vi "Send Image Data.vi"(4 "error in (no error)":errorcluster, 6 "image data":T1, 7 "Response Notifier":string) -> (0 "error out":errorcluster)   [LabVIEW 2020, in "Startup Processes.lvlib"]
uses:
  Startup Processes.lvlib
  <vilib>/picture/picture.llb/imagedata.ctl
  <vilib>/Utility/sysdir.llb/System Directory Type.ctl
  toolbox/Standard Signalling/not_Generic Named Notifier/not_Generic Named Notifier.lvlib
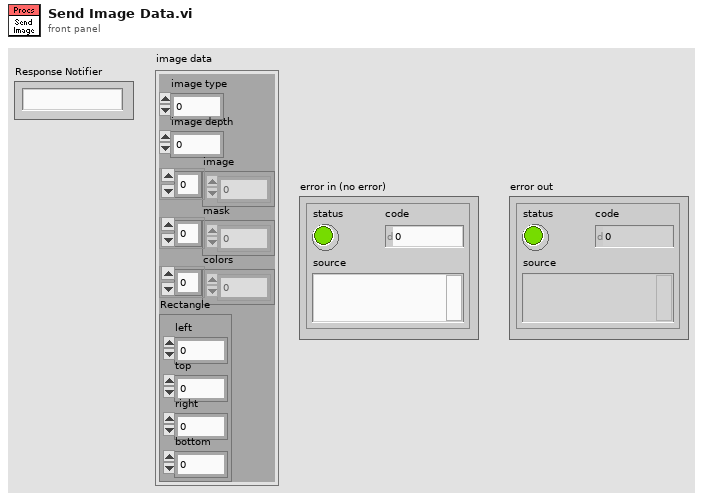
[diagram p1: front panel]
types:
  T1 = typedef "imagedata.ctl" = cluster{"image type":i32, "image depth":i32, "image":u8[], "mask":u8[], "colors":u32[], "Rectangle":cluster{"left":i16, "top":i16, "right":i16, "bottom":i16}}
  T2 = typedef "System Directory Type.ctl" = i32
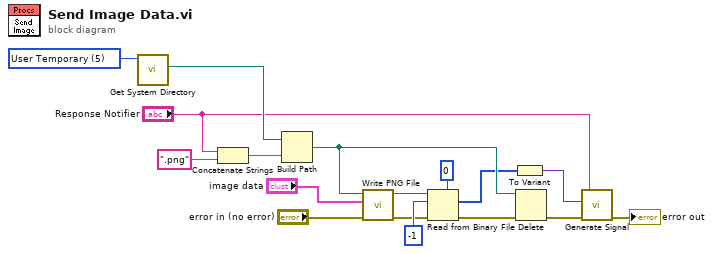
[diagram p0: block diagram]
diagram:
  w16 = T2 5 items=["User Home"=0, "User Desktop"=1, "User Documents"=2, "User Application Data"=3, "User Preferences"=4, "User Temporary"=5, "Public Documents"=6, "Public Application Data"=7, "Public Preferences"=8, "Public Cache"=13, "System Core Libraries"=9, "System Installed Libraries"=10, "Application Files"=11, "Boot Volume Root"=12] ("system directory type")
  n1 = call <vilib>:"Get System Directory.vi"("system directory type"=w16) -> ("system directory"=w17:path)  [unwired: 10 in]
  n2 = Concatenate Strings("Response Notifier", ".png" ("string")) -> (w4:string)
  n3 = Build Path(base path=w17, name or relative path=w4) -> (appended path=w11:path)
  n4 = call <vilib>:"Write PNG File.vi"("error in (no error)"="error in (no error)", "image data"="image data", "path to PNG file"=w11) -> ("error out"=w5:errorcluster, "path"=w6:path)  [unwired: 7 in]
  n5 = Read from Binary File(5:u8 0, 8:w5, 10:-1 ("count (1)"), 11:w6) -> (0:w10:errorcluster, 2:w9:u8[])  [unwired: 2 in, 2 out]
  n6 = To Variant(anything=w9) -> (Variant=w14:variant)
  n7 = Delete(path (use dialog)=w11, error in=w10) -> (error out=w12:errorcluster)  [unwired: 3 in, 2 out]
  n8 = call "Generate Signal.vi"("Error In"=w12, "Signal Data"=w14, "Notifier Name"="Response Notifier") -> ("Error Out"=→"error out":errorcluster)  [unwired: 4 in]
